vi "To-simple-string.vi"(8 "error in (no error)":errorcluster, 11 "Action in":refnum<class "Action.lvclass">) -> (0 "error out":errorcluster, 2 "Action string":string, 3 "Action out":refnum<class "Action.lvclass">)   [LabVIEW 2013, in "PowderDeposition.lvlib" / "Action.lvclass"]
uses:
  Action.lvclass
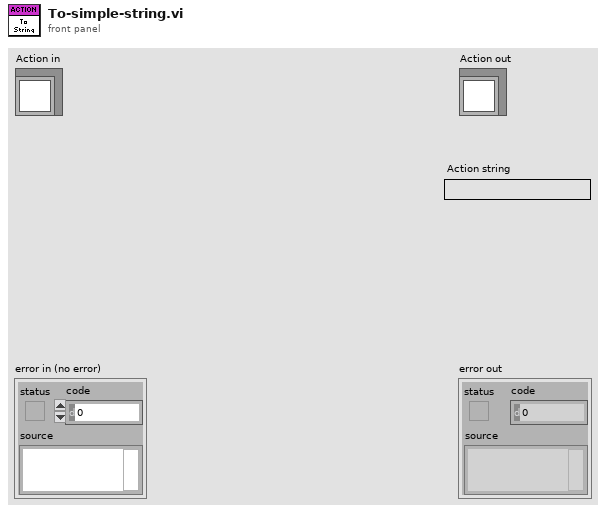
[diagram p1: front panel]
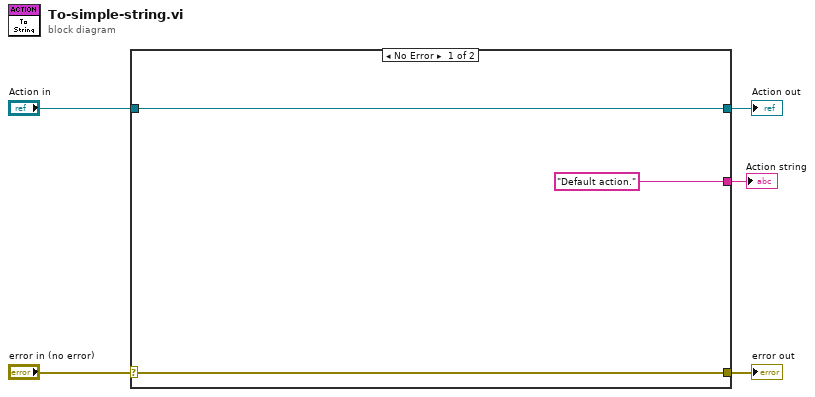
[diagram p0: block diagram]
diagram:
  n1 = case shown="No Error" "error in (no error)" {
    selector: "error in (no error)" -> [w7 w10]
    tunnel: [w7 w10] -> w4
    tunnel: [w8 w9] -> w2
    tunnel: "Action in" -> [w8 w9]
    tunnel: ["Default action." _] -> w1
    frame No Error {
    }
    frame Error {
    }
  }
  "error out" <- w4
  "Action out" <- w2
  "Action string" <- w1
